vi "AgilentLauncher.vi"   [LabVIEW 2014]
uses:
  Project/Implementations/Hardware/Real Hardware/ReadoutDevice/Agilent DSO-X 3032A/Agilent DSO-X 3032A.lvclass
  <vilib>/ActorFramework/Actor/Actor.lvclass
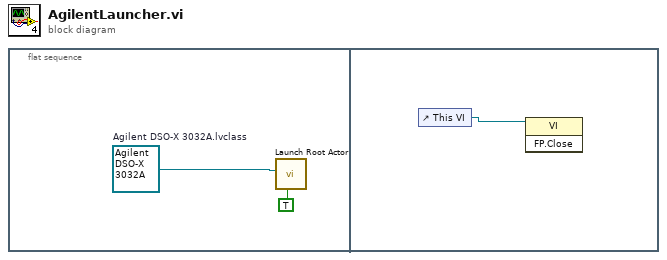
[diagram p0: block diagram]
diagram:
  n1 = flat-sequence {
    frame #0 {
      w1 = refnum<class "Agilent DSO-X 3032A.lvclass"> refnum  # Agilent DSO-X 3032A.lvclass
      n2 = call <vilib>:"Launch Root Actor.vi"("Open Actor Core front panel? (F)"=TRUE, "Actor"=w1) -> ()  [unwired: 8 in, 2 out]
    }
    frame #1 {
      n3 = control-ref of="This VI"() -> (w3:refnum<vi>)
      n4 = invoke class="VI" method="FP.Close"(reference=w3) -> ()  [unwired: 2 in, 3 out]
    }
  }
